vi "sub vi - AI USB4704 (3)  Create Task v3.vi"(0 "Task In 0":dbl, 5 "Task In 1":dbl, 7 "Task In 2":dbl, 9 "Rate Hz":dbl, 11 "Samples":dbl) -> (4 "TASK USB 0":i32, 6 "TASK USB 1":i32, 8 "TASK USB 2":i32, 14 "AI Task Er":bool, 15 "error array":errorcluster[](array[cluster]))   [LabVIEW 2013]
uses:
  <userlib>/DAQNavi Polymorphic VI/create/DAQNavi Create Channel(AI-Voltage).vi
  <userlib>/DAQNavi Polymorphic VI/configure/timing/DAQNavi Timing(Convert Clock).vi
  <userlib>/DAQNavi Polymorphic VI/configure/DAQNavi Get Property/AI/DAQNaviGet_AI_ConvertClock_Rate.vi
panel:
  in  "Tab Control":enum32{"Tasks In", "USB #0", "USB #1", "USB #2"}(tab)
  out "physical channels 0":string="DemoDevice,BID#0/ai0:1" caption="property value"
  out "value range 0":string="+/- 5 V" caption="property value"
  out "convert rate 0":dbl
  out "physical channels 1":string="DemoDevice,BID#0/ai0:1" caption="property value"
  out "value range  1":string="+/- 5 V" caption="property value"
  out "convert rate 1":dbl
  out "physical channels 2":string="DemoDevice,BID#0/ai0:1" caption="property value"
  out "value range  2":string="+/- 5 V" caption="property value"
  out "convert rate 2":dbl
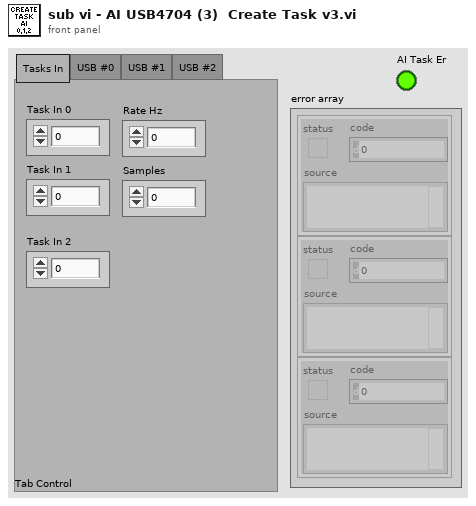
[diagram p1: front panel]
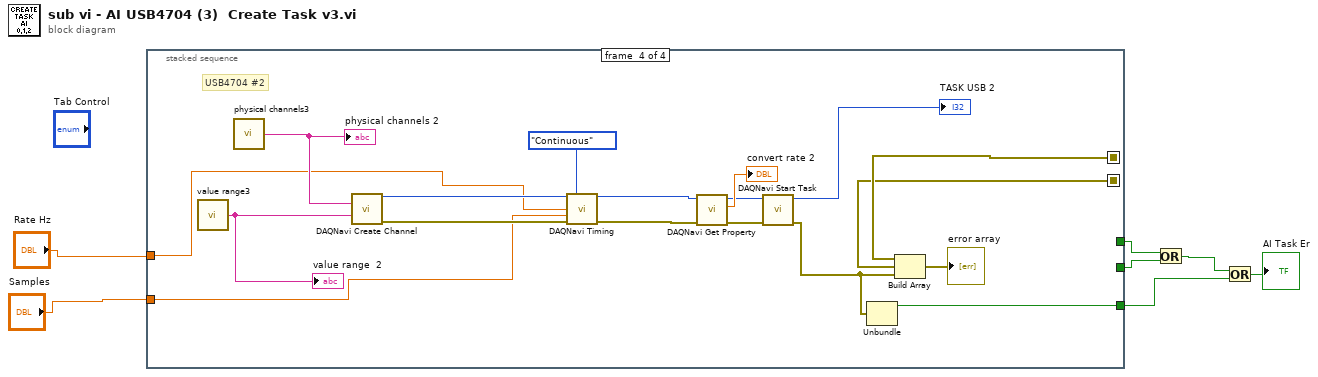
[diagram p0: block diagram]
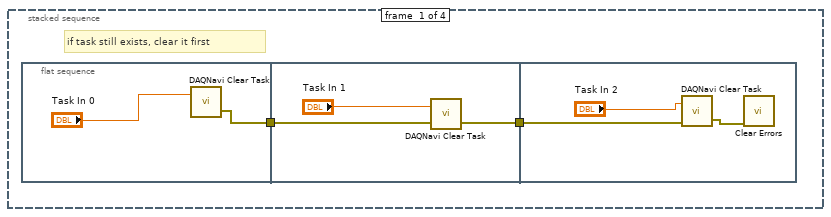
[diagram p2: hidden frame]
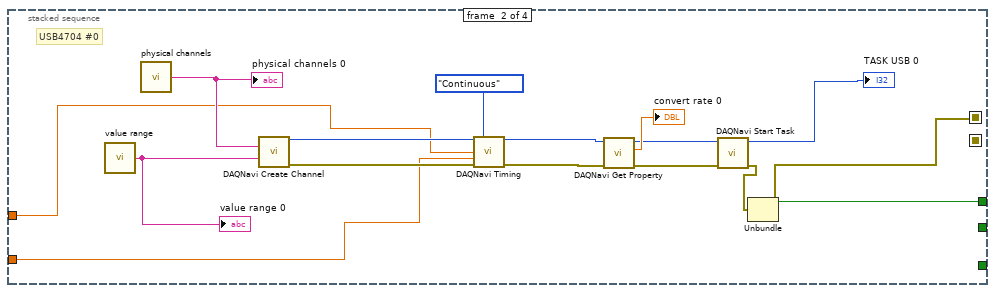
[diagram p3: hidden frame]
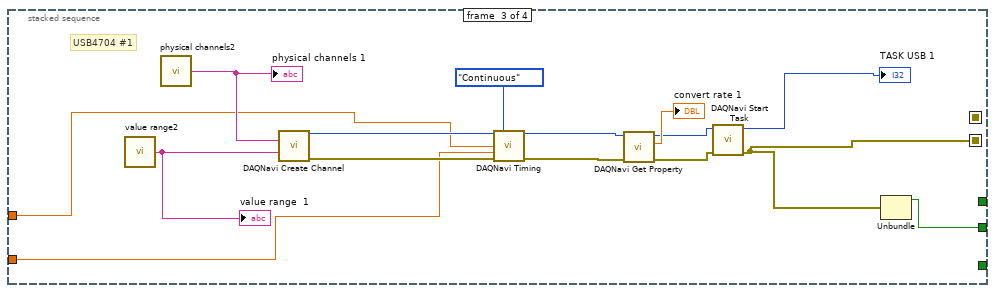
[diagram p4: hidden frame]
diagram:
  n1 = stacked-sequence {
    seq-local: [_ w18 _ _] -> [_ _ _ w57]
    seq-local: [_ _ w34 _] -> [_ _ _ w56]
    tunnel: "Rate Hz" -> [_ w24 w39 w54]
    tunnel: "Samples" -> [_ w23 w38 w53]
    tunnel: [_ _ _ w52] -> w5
    tunnel: [_ w22 _ _] -> w4
    tunnel: [_ _ w37 _] -> w3
    frame #0 {
      # "if task still exists, clear it first"
      n2 = flat-sequence {
        tunnel: [w11] -> w9
        tunnel: w9 -> [w14]
        tunnel: [w13] -> w8
        tunnel: w8 -> [w17]
        frame #0 {
          n3 = call <userlib>:"DAQNavi Clear Task.vi"("task in"="Task In 0") -> ("error out"=w11:errorcluster)  [unwired: 2 in]
        }
        frame #1 {
          n4 = call <userlib>:"DAQNavi Clear Task.vi"("error in (no error)"=w14, "task in"="Task In 1") -> ("error out"=w13:errorcluster)  [unwired: 1 in]
        }
        frame #2 {
          n5 = call <userlib>:"DAQNavi Clear Task.vi"("error in (no error)"=w17, "task in"="Task In 2") -> ("error out"=w16:errorcluster)  [unwired: 1 in]
          n6 = call <vilib>:"Clear Errors.vi"("error in (no error)"=w16) -> ()  [unwired: 6 in, 1 out]
        }
      }
    }
    frame #1 {
      # "USB4704 #0"
      n7 = call "value range"() -> ("property value"=w32:string)  [unwired: 1 out]
      "value range 0" <- w32
      n8 = call "physical channels"() -> ("property value"=w31:string)  [unwired: 1 out]
      "physical channels 0" <- w31
      n9 = call-poly <userlib>:"DAQNavi Create Channel.vi"("physical channels"=w31, "value range"=w32) -> ("task out"=w25:i32, "error out"=w26:errorcluster)  [unwired: 3 in, 9 out]
      n10 = call-poly <userlib>:"DAQNavi Timing.vi"("task in"=w25, "sample mode"=enum16{"Finite", "Continuous"}."Continuous", "rate"=w24, "samples per channel"=w23, "error in (no error)"=w26) -> ("task out"=w28:i32, "error out"=w29:errorcluster)  [unwired: 1 in, 8 out]
      n11 = call-poly <userlib>:"DAQNavi Get Property.vi"("error in (no error)"=w29, "task in"=w28) -> ("error out"=w21:errorcluster, "rate"=→"convert rate 0":dbl, "task out"=w20:i32)  [unwired: 7 out]
      n12 = call <userlib>:"DAQNavi Start Task.vi"("error in (no error)"=w21, "task in"=w20) -> ("error out"=w18:errorcluster, "task out"=→"TASK USB 0":i32)  [unwired: 8 in]
      n13 = Unbundle(w18) -> ("status"=w22:bool)  [unwired: 2 out]
    }
    frame #2 {
      # "USB4704 #1"
      n14 = call "value range2"() -> ("property value"=w47:string)  [unwired: 1 out]
      "value range  1" <- w47
      n15 = call "physical channels2"() -> ("property value"=w46:string)  [unwired: 1 out]
      "physical channels 1" <- w46
      n16 = call-poly <userlib>:"DAQNavi Create Channel.vi"("physical channels"=w46, "value range"=w47) -> ("task out"=w40:i32, "error out"=w41:errorcluster)  [unwired: 3 in, 9 out]
      n17 = call-poly <userlib>:"DAQNavi Timing.vi"("task in"=w40, "sample mode"=enum16{"Finite", "Continuous"}."Continuous", "rate"=w39, "samples per channel"=w38, "error in (no error)"=w41) -> ("task out"=w43:i32, "error out"=w44:errorcluster)  [unwired: 1 in, 8 out]
      n18 = call-poly <userlib>:"DAQNavi Get Property.vi"("error in (no error)"=w44, "task in"=w43) -> ("error out"=w36:errorcluster, "rate"=→"convert rate 1":dbl, "task out"=w35:i32)  [unwired: 7 out]
      n19 = call <userlib>:"DAQNavi Start Task.vi"("error in (no error)"=w36, "task in"=w35) -> ("error out"=w34:errorcluster, "task out"=→"TASK USB 1":i32)  [unwired: 8 in]
      n20 = Unbundle(w34) -> ("status"=w37:bool)  [unwired: 2 out]
    }
    frame #3 {
      # "USB4704 #2"
      n21 = call "value range3"() -> ("property value"=w65:string)  [unwired: 1 out]
      "value range  2" <- w65
      n22 = call "physical channels3"() -> ("property value"=w64:string)  [unwired: 1 out]
      "physical channels 2" <- w64
      n23 = call-poly <userlib>:"DAQNavi Create Channel.vi"("physical channels"=w64, "value range"=w65) -> ("task out"=w58:i32, "error out"=w59:errorcluster)  [unwired: 3 in, 9 out]
      n24 = call-poly <userlib>:"DAQNavi Timing.vi"("task in"=w58, "sample mode"=enum16{"Finite", "Continuous"}."Continuous", "rate"=w54, "samples per channel"=w53, "error in (no error)"=w59) -> ("task out"=w61:i32, "error out"=w62:errorcluster)  [unwired: 1 in, 8 out]
      n25 = call-poly <userlib>:"DAQNavi Get Property.vi"("error in (no error)"=w62, "task in"=w61) -> ("error out"=w50:errorcluster, "rate"=→"convert rate 2":dbl, "task out"=w51:i32)  [unwired: 7 out]
      n26 = call <userlib>:"DAQNavi Start Task.vi"("error in (no error)"=w50, "task in"=w51) -> ("error out"=w49:errorcluster, "task out"=→"TASK USB 2":i32)  [unwired: 8 in]
      n27 = Unbundle(w49) -> ("status"=w52:bool)  [unwired: 2 out]
      n28 = Build Array(w57, w56, w49) -> (→"error array":errorcluster[])
    }
  }
  n29 = Or(x=w4, y=w3) -> (x .or. y?=w6:bool)
  n30 = Or(x=w6, y=w5) -> (x .or. y?=→"AI Task Er":bool)
